vi "TP Buffer Create New TP Connection.vi"(5 "CAN frame":T1 {"payload" format="%x"; "timestamp" format="%<%.7X\n%x>T"; "type" items=["CAN Data"=0, "CAN Remote"=1, "CAN Bus Error"=2, "J1939 Data"=192, "Delay"=224, "Log Trigger"=225, "Start Trigger"=226]; "identifier" format="%x"}, 11 "error in (no error)":errorcluster) -> (4 "Connection Cluster Out":T3, 15 "error out":errorcluster)   [LabVIEW 2013, in "J1939.lvlib"]
uses:
  J1939.lvlib
  TP Buffer Connection Cluster.ctl
  <vilib>/xnet/xnet.llb/XNET Frame CAN.ctl
  <vilib>/xnet/xnet.llb/XNET Frame Type CAN.ctl
  Frame Conversion/Convert CAN Arb ID to J1939 ID.vi
  Frame Conversion/Convert PGN + SA to J1939 ID.vi
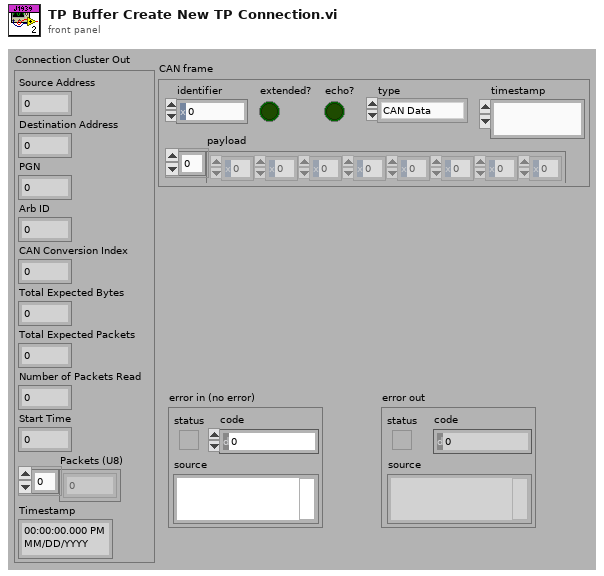
[diagram p1: front panel]
types:
  T1 = typedef "XNET Frame CAN.ctl" = cluster{"timestamp":timestamp, "payload":u8[], "identifier":u32, "type":T2, "extended?":bool, "echo?":bool}
  T2 = typedef "XNET Frame Type CAN.ctl" = u8
  T3 = typedef "J1939.lvlib/TP Buffer Connection Cluster.ctl" = cluster{"Source Address":u8, "Destination Address":u8, "PGN":u32, "Arb ID":u32, "CAN Conversion Index":u32, "Total Expected Bytes":u16, "Total Expected Packets":u8, "Number of Packets Read":u8, "Start Time":u32, "Packets (U8)":u8[], "Timestamp":timestamp}
  T4 = typedef "J1939.lvlib/PGN Fields Cluster.ctl" = cluster{"Reserved Bit":u8, "Data page":u8, "PDU Format":u8, "PDU Specific":u8}
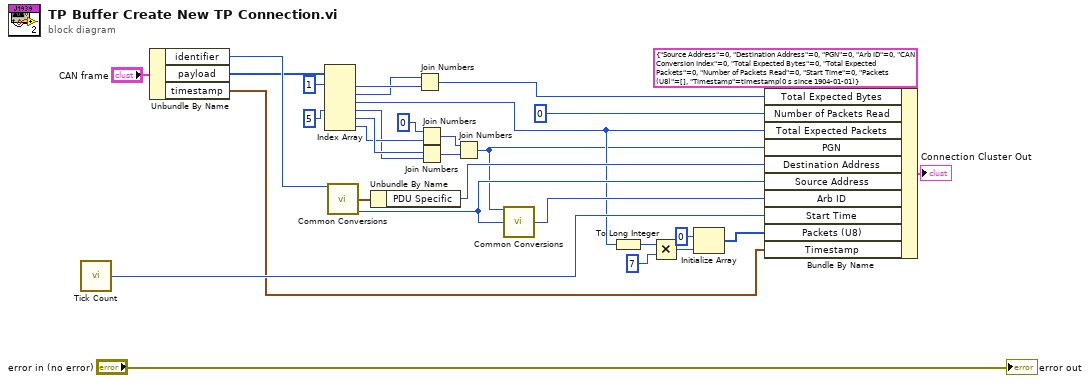
[diagram p0: block diagram]
diagram:
  n1 = call "Tick Count"() -> ("Tick Count(mSec)"=w31:u32)
  n2 = Unbundle By Name("CAN frame") -> ("identifier"=w20:u32, "payload"=w19:u8[], "timestamp"=w9:timestamp)
  n3 = Index Array(array=w19, index #1=1 ("index"), index #4=5 ("index")) -> (element #1=w6:u8, element #2=w5:u8, element #3=w18:u8, element #4=w2:u8, element #5=w16:u8, element #6=w3:u8)  [unwired: 4 in]
  n4 = call-poly "Common Conversions.vi"("Arb ID"=w20) -> ("PGN Fields"=w29:T4, "Source Address"=w26:u8)  [unwired: 13 out]
  n5 = Unbundle By Name(w29) -> ("PDU Specific"=w27:u8)
  n6 = Join Numbers(hi=w5, lo=w6) -> ((hi.lo)=w10:u16)
  n7 = Join Numbers(hi=u8 0, lo=w3) -> ((hi.lo)=w15:u16)
  n8 = Join Numbers(hi=w16, lo=w2) -> ((hi.lo)=w14:u16)
  n9 = Join Numbers(hi=w15, lo=w14) -> ((hi.lo)=w13:u32)
  n10 = call-poly "Common Conversions.vi"("PGN"=w13, "Source Address"=w26) -> ("ARB ID"=w25:u32)  [unwired: 2 in, 11 out]
  n11 = To Long Integer(number=w18) -> (32bit integer=w4:i32)
  n12 = Multiply(x=w4, y=7 ("x")) -> (x*y=w22:i32)
  n13 = Initialize Array(u8 0 ("element"), w22) -> (w23:u8[])
  n14 = Bundle By Name(cluster=T3 {"Source Address"=0, "Destination Address"=0, "PGN"=0, "Arb ID"=0, "CAN Conversion Index"=0, "Total Expected Bytes"=0, "Total Expected Packets"=0, "Number of Packets Read"=0, "Start Time"=0, "Packets (U8)"=[], "Timestamp"=timestamp(0 s since 1904-01-01)} ("Connection Cluster"), "Total Expected Bytes"=w10, "Number of Packets Read"=u8 0, "Total Expected Packets"=w18, "PGN"=w13, "Destination Address"=w27, "Source Address"=w26, "Arb ID"=w25, "Start Time"=w31, "Packets (U8)"=w23, "Timestamp"=w9) -> (→"Connection Cluster Out":T3)
  "error out" <- "error in (no error)"
